vi "DN4_2DarrayTo1Darray.vi"(3 "error in (no error)":errorcluster, 4 "samples":i32, 5 "channel count":i32, 6 "2Darray":dbl[][](array[numeric])) -> (0 "error out":errorcluster, 2 "1Darray":dbl[](array[numeric]))   [LabVIEW 2009]
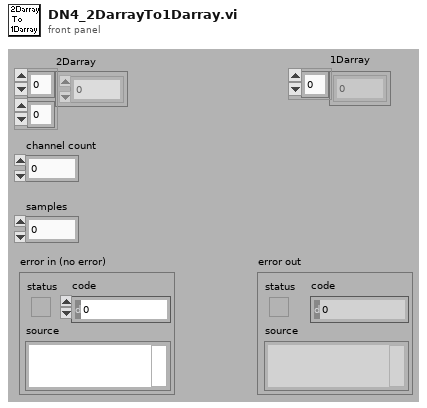
[diagram p1: front panel]
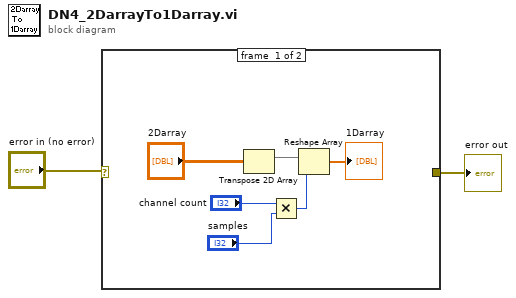
[diagram p0: block diagram]
diagram:
  n1 = case shown="No Error" "error in (no error)" {
    selector: "error in (no error)" -> [_ w9]
    tunnel: [_ w9] -> w1
    frame #0 {
      n2 = Transpose 2D Array(2D array="2Darray") -> (transposed array=w8:dbl[][])
      n3 = Multiply(x="channel count", y="samples") -> (x*y=w7:i32)
      n4 = Reshape Array(w8, w7) -> (→"1Darray":dbl[])
    }
    frame #1 {
    }
  }
  "error out" <- w1
